vi "pid-positionControl.vi"() -> ()   [LabVIEW 2011]
uses:
  <vilib>/Simulation/Scripting/Companion Diagram/SimConfigNode/SimParams.ctl
  <vilib>/Simulation/Scripting/Companion Diagram/SimConfigNode/_simSolvers.ctl
  <vilib>/Simulation/Implementation/Shared/SIMSCR Execution Mode.ctl
  <vilib>/Simulation/Param Hierarchy/Typedefs/SIMPH Param Control Actions.ctl
  <vilib>/MakerHub/LINX/Public/Peripherals/Analog/Analog Read 1 Chan.vi
  <vilib>/Simulation/Implementation/Shared/NILVSim_FinalizeModel.vi
  <vilib>/Simulation/Implementation/Shared/NILVSim_Manager.vi
  <vilib>/Simulation/Implementation/Shared/NILVSim_ParamChanged.vi
  <vilib>/MakerHub/LINX/Public/Peripherals/PWM/PWM Set Duty Cycle 1 Chan.vi
  <vilib>/MakerHub/LINX/Public/Peripherals/Analog/Analog Read N Chans.vi
  <vilib>/MakerHub/LINX/Private/Local IO/LinxAnalogRead.vi
  <vilib>/MakerHub/LINX/Public/Utilities/Check Channel.vi
  <vilib>/MakerHub/LINX/Public/Utilities/Open Serial.vi
  <vilib>/MakerHub/LINX/Private/Utilties/Generate Error.vi
  <vilib>/Simulation/Implementation/Shared/SIM Unbundle Sim Info.vi
  <vilib>/Simulation/Implementation/Shared/NILVSim_GetModelError.vi
  <vilib>/Simulation/Implementation/Shared/SIM Bundle Sim Info.vi
  <vilib>/Simulation/Implementation/Shared/NILVSim_Initialize.vi
  <vilib>/MakerHub/LINX/Public/Peripherals/PWM/PWM Set Duty Cycle N Chans.vi
  <vilib>/Simulation/Implementation/XNodeFramework/SimXNode/SimX.xnode
  <vilib>/Simulation/Model Libraries/PID/SIM PID (Academic).vi
  <vilib>/Simulation/Model Libraries/PID/SIM PID.vi
  <vilib>/Simulation/Scripting/Companion Diagram/SimConfigNode/SimDog.xnode
  <vilib>/MakerHub/LINX/LMH-LINX.lvlib
  <vilib>/Simulation/Implementation/Shared/NI_SIM_Implementation.lvlib
panel:
  out "PID Output":dbl
  out "SetPoint":dbl(knob) scale=0.0..180.0 scale format="%#_11g"
  out "Angulo":dbl
  out "Angulo Atual":dbl(knob) scale=0.0..180.0 scale format="%#_11g"
  out "PID":dbl
  in  "Derivative time [s] (Td)":dbl=1.0
  in  "Integral time [s] (Ti)":dbl=1.0
  in  "Proportional Gain (Kc)":dbl=1.0
  in  "stop":bool
  in  "SetPoint":dbl format="%.2f"
  in  "Serial Port":refnum<visa-resource-name>="N/A"
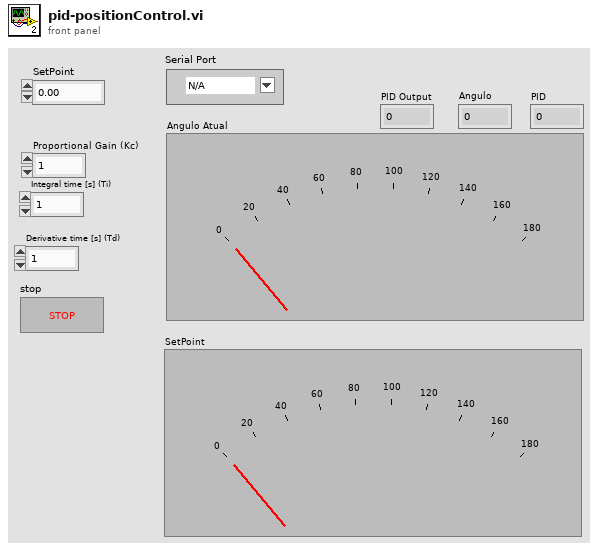
[diagram p1: front panel]
types:
  T1 = enum16{"open", "replace", "create", "open or create", "replace or create", "replace or create with confirmation"}
  T2 = typedef "SIMPH Param Control Actions.ctl" = enum16{"get params", "set params"}
  T3 = typedef "SimParams.ctl" = cluster{"Initial Time (s)":dbl, "Final Time (s)":dbl, "Step Size (s)":dbl, "ODE Solver":T4, "Minimum Step Size (s)":dbl, "Maximum Step Size (s)":dbl, "Relative Tolerance":dbl, "Absolute Tolerance":dbl, "Software Timing":bool, "Initial Step Size (s)":dbl, "Automatic Fixed Step Size?":bool, "Automatic Discrete Step Size?":bool, "Discrete Step Size (s)":dbl, "Calculate using Time Step":bool, "Solver Wired?":bool, "Prev.Frm.Expected End":u64, "Prev.Frm.Actual End":u64, "Prev.Frm.Finished Late?":bool, "Prev.Iter.Expected End":u64, "Prev.Iter.Actual End":u64, "Prev.Iter.Finished Late?":bool, "Expected Iteration Start":u64, "Actual Iteration Start":u64, "Expected Frame Start":u64, "Actual Frame Start":u64, "Source Name":string, "Name":string, "Period":i64, "Deadline":i64, "Offset":i64, "Start":i64, "Priority":i32, "Timeout":i32, "Processor":i32, "Mode":enum32{"No Change", "Process missed periods, maintain original phase", "Discard missed periods, maintain original phase", "Process missed periods, ignore original phase", "Discard missed periods, ignore original phase"}, "Wakeup reason":enum32{"Normal", "Aborted", "Asynchronous wakeup", "Timing source error", "Timed loop error", "Timeout"}, "Error":errorcluster, "Source Type":string, "Secondary Source Type":string, "Global End Time":u64, "Global Start Time":u64, "Full Solver Reset":bool, "Execution Mode":T5, "Nan/Inf Check":bool, "Custom Solver Library":string, "Solver Is Variable":bool, "custom solver name":string}
  T4 = typedef "_simSolvers.ctl" = enum16{"Runge-Kutta 1 (Euler)", "Runge-Kutta 2", "Runge-Kutta 3", "Runge-Kutta 4", "Runge-Kutta 23 (variable)", "Runge-Kutta 45 (variable)", "BDF (variable)", "Adams-Moulton (variable)", "Rosenbrock (variable)", "Discrete States Only", "Linearizer", "State Query", "Trim Eval", "Custom Solver"}
  T5 = typedef "SIMSCR Execution Mode.ctl" = u16
  T6 = typedef "LMH-LINX.lvlib/LINX Ref.ctl" = cluster{"IO":T7, "Interface":T8, "LINX Device Config":T9}
  T7 = typedef "LMH-LINX.lvlib/Platform.ctl" = enum16{"Remote", "Local"}
  T8 = typedef "LMH-LINX.lvlib/Interface.ctl" = enum16{"Serial", "TCP"}
  T9 = typedef "LMH-LINX.lvlib/Device.lvlib/LINX Device Config.ctl" = cluster{"Interface":T8, "COM Port":refnum<visa-resource-name>, "TCP Configuration":T10, "Device Family":u8, "Device ID":u8, "Device Name":string, "TCP Ref":refnum<k5>, "Channels":T11}
  T10 = typedef "LMH-LINX.lvlib/Device.lvlib/TCP Config.ctl" = cluster{"IP Address":string, "Port":u16}
  T11 = typedef "LMH-LINX.lvlib/Channels.ctl" = cluster{"DI":u8[], "DO":u8[], "AI":u8[], "AO":u8[], "PWM":u8[], "QE":u8[], "UART":u8[], "I2C 2":u8[], "SPI":u8[], "CAN":u8[], "Servo":u8[], "AI Ref (V)":dbl, "AI Resolution (Bits)":u8, "AO Ref (V)":dbl, "AO Resolution (Bits)":u8}
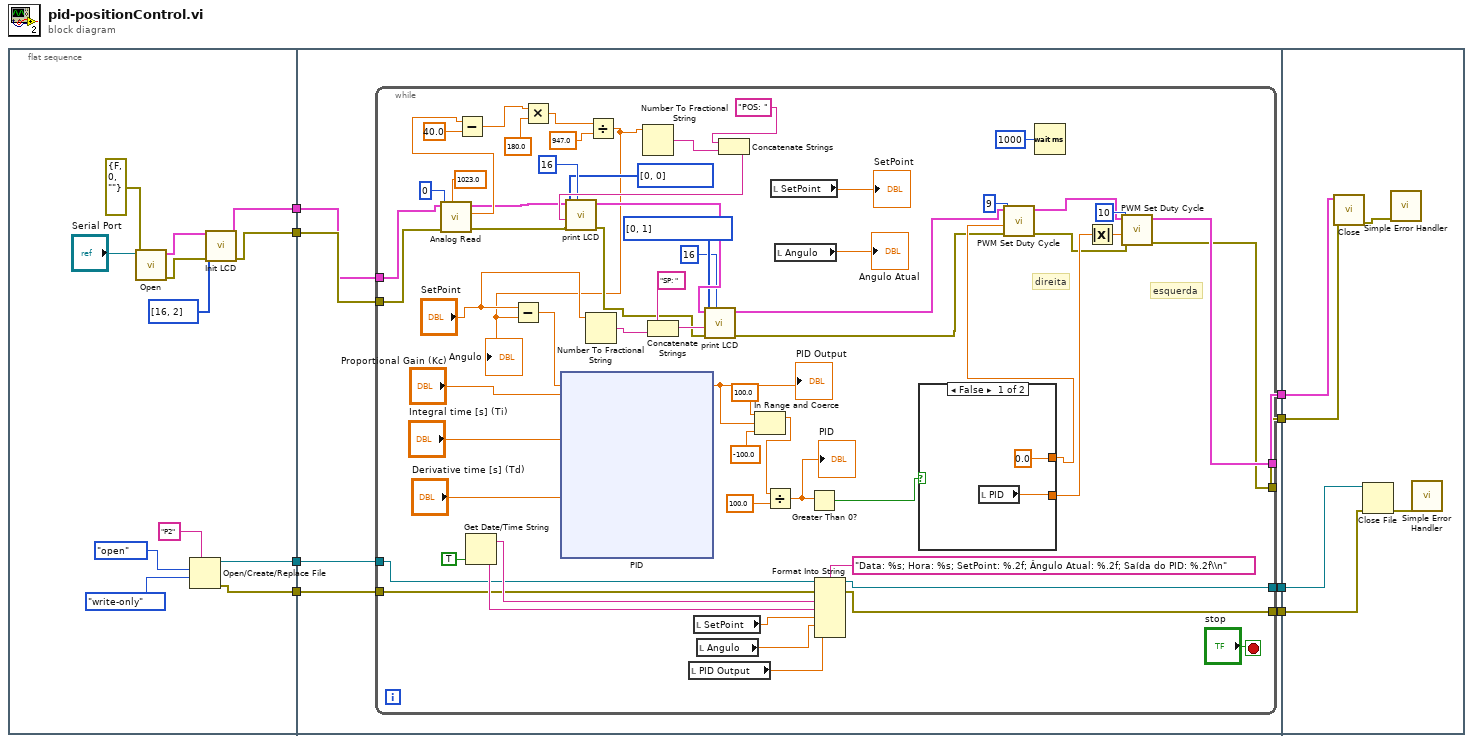
[diagram p0: block diagram]
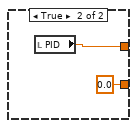
[diagram p2: hidden frame]
diagram:
  n1 = flat-sequence {
    tunnel: [w16] -> w8
    tunnel: [w15] -> w7
    tunnel: [w10] -> w4
    tunnel: [w9] -> w1
    tunnel: w8 -> [w28]
    tunnel: w7 -> [w27]
    tunnel: [w26] -> w6
    tunnel: [w25] -> w5
    tunnel: w4 -> [w24]
    tunnel: [w23] -> w3
    tunnel: [w22] -> w2
    tunnel: w1 -> [w21]
    tunnel: w6 -> [w229]
    tunnel: w5 -> [w228]
    tunnel: w3 -> [w226]
    tunnel: w2 -> [w225]
    frame #0 {
      n2 = call-poly <vilib>:"Open.vi"("Error In"=errorcluster {"status"=FALSE, "code"=0, "source"=""}, "Serial Port"="Serial Port") -> ("Error Out"=w20:errorcluster, "LINX Resource"=w19:T6)  [unwired: 7 in, 1 out]
      n3 = Open/Create/Replace File(prompt="P2", operation (0:open)=T1."open", access (0:read/write)=enum16{"read/write", "read-only", "write-only"}."write-only") -> (refnum out=w10:refnum<file>, error out=w9:errorcluster)  [unwired: 3 in, 1 out]
      n4 = call "Init LCD.vi"("LINX Resource"=w19, "Colunas/Linhas"=u8[] [16, 2], "Error In"=w20) -> ("LINX Resource 2"=w15:T6, "Error Out"=w16:errorcluster)  [unwired: 11 in]
    }
    frame #1 {
      n5 = while {
        tunnel: w28 -> [w41]
        tunnel: w27 -> [w42]
        tunnel: [w47] -> w26
        tunnel: [w46] -> w25
        tunnel: w24 -> [w38]
        tunnel: [w37] -> w23
        tunnel: [w36] -> w22
        tunnel: w21 -> [w35]
        stop <- "stop" stop-if-true
        # "esquerda"
        # "direita"
        n6 = call-poly <vilib>:"Analog Read.vi"("Analog Ref Override (V)"=1023.0, "Error In"=w41, "Analog Channel"=u8 0, "LINX Resource"=w42) -> ("Error Out"=w59:errorcluster, "Voltage"=w85:dbl, "LINX Resource"=w60:T6)  [unwired: 4 in, 1 out]
        n7 = Subtract(x=w85, y=40.0) -> (x-y=w83:dbl)
        n8 = Get Date/Time String(want seconds? (F)=TRUE) -> (date string=w40:string, time string=w39:string)  [unwired: 2 in]
        n9 = Multiply(x=w83, y=180.0) -> (x*y=w81:dbl)
        n10 = Number To Fractional String(number="SetPoint") -> (F-format string=w72:string)  [unwired: 3 in]
        n11 = Divide(x=w81, y=947.0) -> (x/y=w45:dbl)
        "Angulo" <- w45
        n12 = Subtract(x="SetPoint", y=w45) -> (x-y=w58:dbl)
        n13 = xnode "PID"("Error"=w58, "Proportional Gain (Kc)"="Proportional Gain (Kc)", "Integral time [s] (Ti)"="Integral time [s] (Ti)", "Derivative time [s] (Td)"="Derivative time [s] (Td)") -> ("Output"=w79:dbl)  [unwired: 2 in, 11 out]
        "PID Output" <- w79
        n14 = Number To Fractional String(number=w45) -> (F-format string=w70:string)  [unwired: 3 in]
        n15 = Concatenate Strings("SP: " ("string"), w72) -> (w68:string)
        n16 = local read "PID Output"() -> (w32:dbl)
        n17 = local read "SetPoint"() -> (w34:dbl)
        n18 = local read "Angulo"() -> (w33:dbl)
        n19 = Concatenate Strings("POS: " ("concatenated string"), w70) -> (w73:string)
        n20 = call "print LCD.vi"("Numero de colunas"=16, "Error In"=w59, "Texto"=w73, "Coluna/linha"=u8[] [0, 0], "LINX Resource"=w60) -> ("Error Out"=w66:errorcluster, "LINX Resource 2"=w67:T6)  [unwired: 5 in]
        n21 = call "print LCD.vi"("Numero de colunas"=16, "Error In"=w66, "Texto"=w68, "Coluna/linha"=u8[] [0, 1], "LINX Resource"=w67) -> ("Error Out"=w50:errorcluster, "LINX Resource 2"=w51:T6)  [unwired: 5 in]
        n22 = In Range and Coerce(upper limit=100.0, x=w79, lower limit=-100.0) -> (coerced(x)=w76:dbl)  [unwired: 1 out]
        n23 = Divide(x=w76, y=100.0) -> (x/y=w65:dbl)
        "PID" <- w65
        n24 = local read "SetPoint"() -> (→"SetPoint":dbl)
        n25 = local read "Angulo"() -> (→"Angulo Atual":dbl)
        n26 = Greater Than 0?(x=w65) -> (x > 0?=w74:bool)
        n27 = Format Into String(format string="Data: %s; Hora: %s; SetPoint: %.2f; Ângulo Atual: %.2f; Saída do PID: %.2f\\n", initial string=w38, error in=w35, w40, w39, w34, w33, w32) -> (resulting string=w37:refnum<file>, error out=w36:errorcluster)
        n28 = case shown="False" w74 {
          tunnel: [0.0 ("y") w95] -> w52
          tunnel: [w92 0.0 ("y")] -> w53
          frame False {
            n29 = local read "PID"() -> (w92:dbl)
          }
          frame True {
            n30 = local read "PID"() -> (w95:dbl)
          }
        }
        n31 = call-poly <vilib>:"PWM Set Duty Cycle.vi"("Error In"=w50, "Duty Cycle (0-1)"=w52, "PWM Channel"=u8 9, "LINX Resource"=w51) -> ("Error Out"=w48:errorcluster, "LINX Resource"=w49:T6)  [unwired: 6 in]
        n32 = Wait (ms)(milliseconds to wait=u32 1000) -> ()  [unwired: 1 out]
        n33 = Absolute Value(x=w53) -> (abs(x)=w55:dbl)
        n34 = call-poly <vilib>:"PWM Set Duty Cycle.vi"("Error In"=w48, "Duty Cycle (0-1)"=w55, "PWM Channel"=u8 10, "LINX Resource"=w49) -> ("Error Out"=w46:errorcluster, "LINX Resource"=w47:T6)  [unwired: 6 in]
      }
    }
    frame #2 {
      n35 = call <vilib>:"Close.vi"("Error In"=w228, "LINX Resource"=w229) -> ("Error Out"=w227:errorcluster)  [unwired: 9 in]
      n36 = Close File(refnum=w226, error in=w225) -> (error out=w224:errorcluster)  [unwired: 1 out]
      n37 = call <vilib>:"Simple Error Handler.vi"("error in (no error)"=w227) -> ()  [unwired: 4 in, 5 out]
      n38 = call <vilib>:"Simple Error Handler.vi"("error in (no error)"=w224) -> ()  [unwired: 4 in, 5 out]
    }
  }
